vi "BRig_dataLC_ENL_First_DelayOpt_l1.vi"() -> (2 "output_ENL_First_DelayOpt":i32)   [LabVIEW 2014]
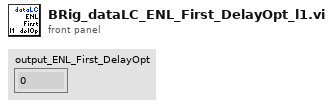
[diagram p1: front panel]
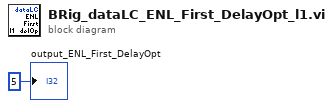
[diagram p0: block diagram]
diagram:
  "output_ENL_First_DelayOpt" <- 5 ("output_iBlock")
